vi "Tell Init Parent.vi"(7 "Actor in":refnum<class "Actor.lvclass">, 9 "Msg":T1 {"Teller"."Absolute Time" format="%<%x %.3X>T"}) -> (0 "Error out":errorcluster, 5 "Actor out":refnum<class "Actor.lvclass">)   [LabVIEW 2020, in "jettl.lvlib"]
uses:
  jettl.lvlib
  Msg/Msg.lvclass
  Msg Contents/Msg Contents.lvclass
  Actor/Actor.lvclass
  Unified Actor Relation.ctl
  Teller.ctl
  Msg.ctl
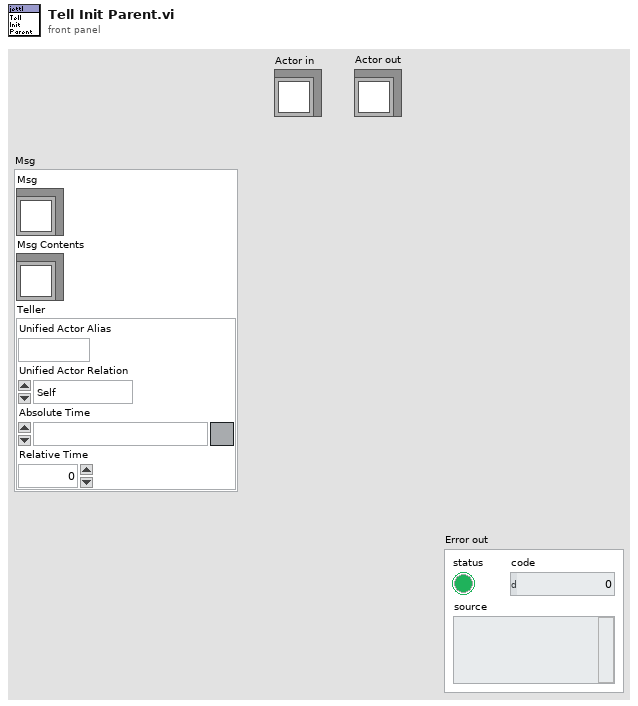
[diagram p1: front panel]
types:
  T1 = typedef "jettl.lvlib/Msg.ctl" = cluster{"Msg":refnum<class "Msg.lvclass">, "Msg Contents":refnum<class "Msg Contents.lvclass">, "Teller":T2}
  T2 = typedef "jettl.lvlib/Teller.ctl" = cluster{"Unified Actor Alias":string, "Unified Actor Relation":T3, "Absolute Time":timestamp, "Relative Time":dbl}
  T3 = typedef "jettl.lvlib/Unified Actor Relation.ctl" = enum16{"Self", "Parent", "Child"}
  T4 = typedef "jettl.lvlib/Unified Actor.ctl" = cluster{"Msgs":T5, "Leaf":bool, "Edge Actors":refnum<class "Actor.lvclass">[], "Mid Actors":refnum<class "Actor.lvclass">[], "Core Actors":refnum<class "Actor.lvclass">[], "Root":bool, "Alias":string, "UID":i32, "Transport":refnum<user-event>, "Address":refnum<event-registration>, "This VI":refnum<vi>}
  T5 = typedef "jettl.lvlib/Msgs.ctl" = cluster{"Inbound":T6, "Outbound":T6, "Implemented":T6, "Tell Init":T6, "Tell Init Self":T6, "Tell Init Parent":T6, "Tell Init Child":T6, "Tell Forward":T6, "Tell Forward Self":T6, "Tell Forward Parent":T6, "Tell Forward Child":T6}
  T6 = typedef "jettl.lvlib/Msg Set.ctl" = set{refnum<class "Msg.lvclass">}
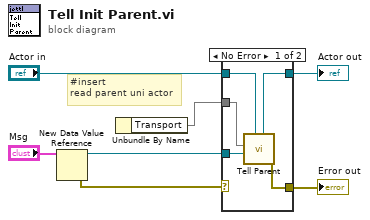
[diagram p0: block diagram]
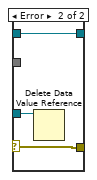
[diagram p2: hidden frame]
diagram:
  # "#insert\nread parent uni actor"
  n1 = New Data Value Reference(data value="Msg") -> (data value reference=w8:refnum<data-value>, error out=w7:errorcluster)  [unwired: 1 in]
  n2 = Unbundle By Name() -> (w2:T4, "Transport"=w1)
  n3 = case shown="No Error" w7 {
    selector: w7 -> [_ w16]
    tunnel: w8 -> [w11 w15]
    tunnel: [w10 w16] -> w4
    tunnel: "Actor in" -> [w13 w14]
    tunnel: [w12 w14] -> w5
    tunnel: w1 -> [w9 _]
    frame No Error {
      n4 = call "Tell Parent.vi"("Actor in"=w13, "Msg DVR"=w11, "Transport"=w9) -> ("Error out"=w10:errorcluster, "Actor out"=w12:refnum<class "Actor.lvclass">)  [unwired: 7 in]
    }
    frame Error {
      n5 = Delete Data Value Reference(data value reference=w15) -> ()  [unwired: 1 in, 2 out]
    }
  }
  "Error out" <- w4
  "Actor out" <- w5
